vi "setId.vi"(8 "error in (no error)":errorcluster, 10 "ID":i32, 11 "pShape in":refnum<class "pShape.lvclass">) -> (0 "error out":errorcluster, 3 "pShape out":refnum<class "pShape.lvclass">)   [LabVIEW 2017, in "pShape.lvclass"]
uses:
  pShape.lvclass
  pShape.lvclass/pShape.ctl
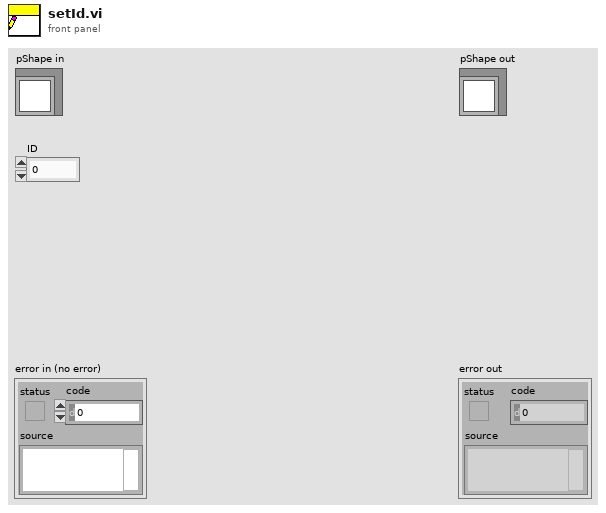
[diagram p1: front panel]
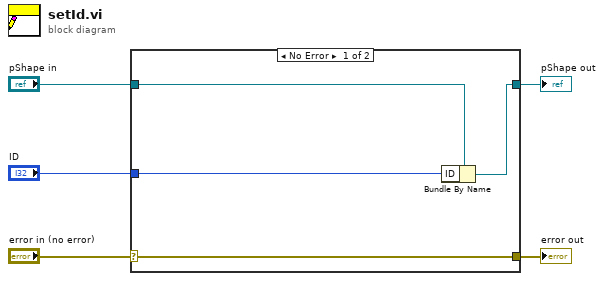
[diagram p0: block diagram]
diagram:
  n1 = case shown="No Error" "error in (no error)" {
    selector: "error in (no error)" -> [w9 w10]
    tunnel: [w9 w10] -> w4
    tunnel: [w7 w11] -> w2
    tunnel: "pShape in" -> [w8 w11]
    tunnel: "ID" -> [w6 _]
    frame No Error {
      n2 = Bundle By Name(cluster=w8, "ID"=w6) -> (w7:refnum<class "pShape.lvclass">)
    }
    frame Error {
    }
  }
  "error out" <- w4
  "pShape out" <- w2
